vi "Init Process.vi"(8 "error in (no error)":errorcluster, 11 "DAQProc in":refnum<class "DAQProc.lvclass">) -> (0 "error out":errorcluster, 3 "DAQProc out":refnum<class "DAQProc.lvclass">)   [LabVIEW 2020, in "LAF2024Q2.lvlib" / "DAQProc.lvclass"]
uses:
  DAQProc.lvclass
  DAQProc.lvclass/DAQProc.ctl
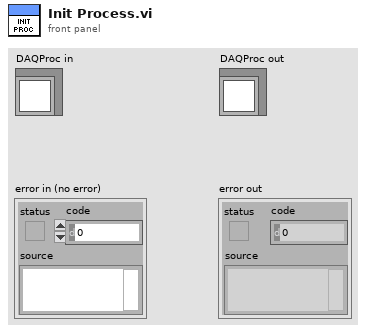
[diagram p1: front panel]
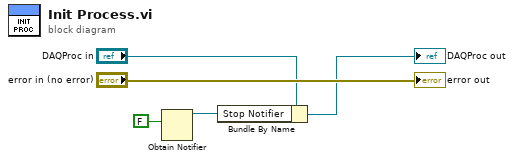
[diagram p0: block diagram]
diagram:
  n1 = Obtain Notifier(notification data type=FALSE) -> (notifier out=w1:refnum<notifier>)  [unwired: 3 in, 2 out]
  n2 = Bundle By Name(cluster="DAQProc in", "Stop Notifier"=w1) -> (→"DAQProc out":refnum<class "DAQProc.lvclass">)
  "error out" <- "error in (no error)"
